vi "Write Context I32.vi"(8 "error in (no error)":errorcluster, 10 "Context I32":i32, 11 "Context Actor in":refnum<class "Context.lvclass">) -> (0 "error out":errorcluster, 3 "Context Actor out":refnum<class "Context.lvclass">)   [LabVIEW 2021, in "Context.lvlib" / "Context.lvclass"]
uses:
  Context.lvclass
  Context.lvclass/Context.ctl
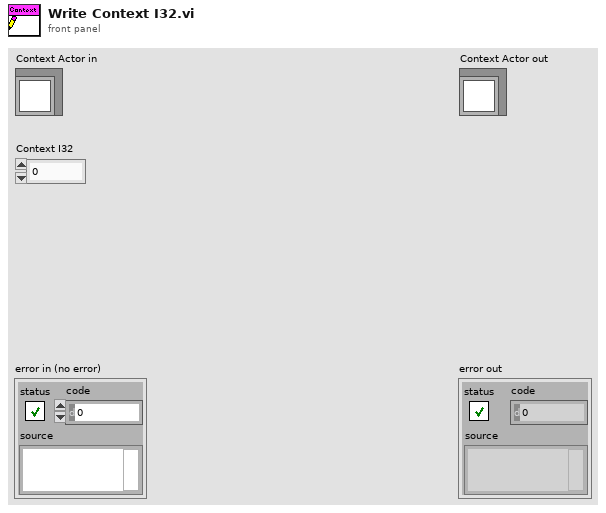
[diagram p1: front panel]
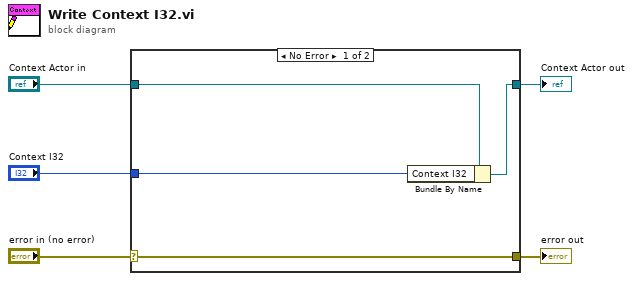
[diagram p0: block diagram]
diagram:
  n1 = case shown="No Error" "error in (no error)" {
    selector: "error in (no error)" -> [w9 w10]
    tunnel: [w9 w10] -> w4
    tunnel: [w7 w11] -> w2
    tunnel: "Context Actor in" -> [w8 w11]
    tunnel: "Context I32" -> [w6 _]
    frame No Error {
      n2 = Bundle By Name(cluster=w8, "Context I32"=w6) -> (w7:refnum<class "Context.lvclass">)
    }
    frame Error {
    }
  }
  "error out" <- w4
  "Context Actor out" <- w2
